vi "CurrentMeas.vi"(8 "error in (no error)":errorcluster, 9 "DxSupply":string="0", 10 "Measure Record Length":i32=5, 11 "instrument handle":refnum<k15>) -> (0 "error out":errorcluster, 1 "Idd Peak":dbl, 2 "Idd Average":dbl format="%0.2f", 3 "instrument handle out":refnum<k15>)   [LabVIEW 2018]
uses:
  <instrlib>/niDCPower/nidcpower.llb/niDCPower Measurement Type.ctl
  <vilib>/Analysis/baseanly.llb/Mean (DBL).vi
  <vilib>/Analysis/NI_AALBase.lvlib
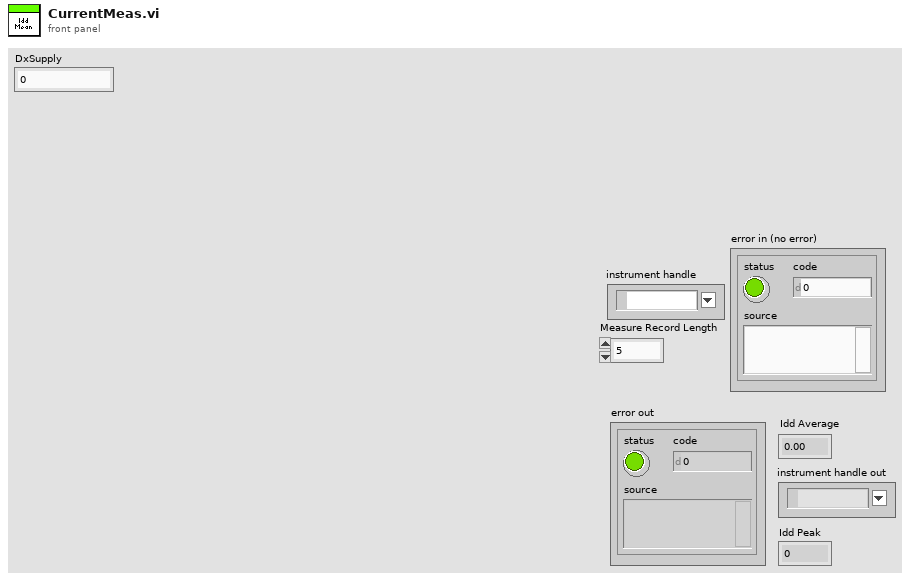
[diagram p1: front panel]
types:
  T1 = typedef "niDCPower Measurement Type.ctl" = i32
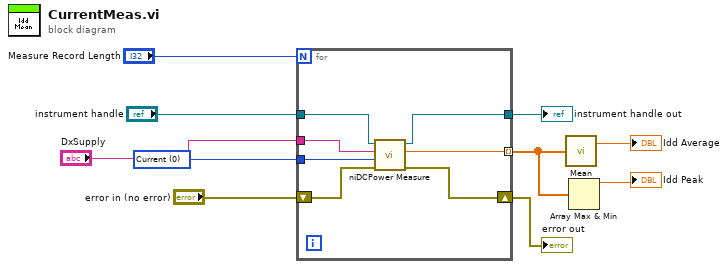
[diagram p0: block diagram]
diagram:
  w10 = T1 0 items=["Current", "Voltage"] ("measurement type")
  n1 = for {
    N: "Measure Record Length" -> [_]
    tunnel: w10 -> [w17]
    tunnel: [w14] -> w2 mode=indexing
    tunnel: "DxSupply" -> [w12]
    shift-right: [w15] -> w8
    shift-left: "error in (no error)" -> [w16]
    tunnel: "instrument handle" -> [w11]
    tunnel: [w13] -> w7
    n2 = call <instrlib>:"niDCPower Measure.vi"("error in (no error)"=w16, "measurement type"=w17, "channel name"=w12, "instrument handle"=w11) -> ("error out"=w15:errorcluster, "measurement"=w14:dbl, "instrument handle out"=w13:refnum<k15>)  [unwired: 5 in]
  }
  "error out" <- w8
  "instrument handle out" <- w7
  n3 = call-poly <vilib>:"Mean.vi"("X"=w2) -> ("mean"=→"Idd Average":dbl)  [unwired: 1 out]
  n4 = Array Max & Min(array=w2) -> (max value=→"Idd Peak":dbl)  [unwired: 3 out]
